vi "writeToXML.vi"(8 "error in (no error)":errorcluster, 10 "Class Label":string="WavefrontTargetPosition", 11 "WaveFrontTargetPosition in":refnum<class "WaveFrontTargetPosition.lvclass">) -> (0 "error out":errorcluster, 2 "XMLout":string, 3 "WaveFrontTargetPosition out":refnum<class "WaveFrontTargetPosition.lvclass">)   [LabVIEW 2022 SP3, in "TCSDataDefinitions.lvlib" / "TCSWFSStatus.lvlib" / "WaveFrontTargetPosition.lvclass"]
uses:
  WaveFrontTargetPosition.lvclass
  WaveFrontTargetPosition.lvclass/WaveFrontTargetPosition.ctl
  TCSWFSStatus/TCSWFSStatus.lvclass
  TCSGuiderStatus/GWTargetPositionParameters/GWTargetPositionParameters.lvclass
  <userlib>/Common/XML/XMLGenerator/XMLGenerator.lvclass
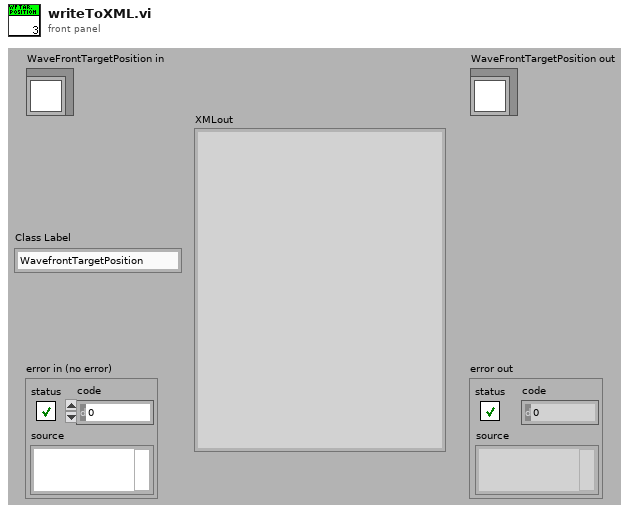
[diagram p1: front panel]
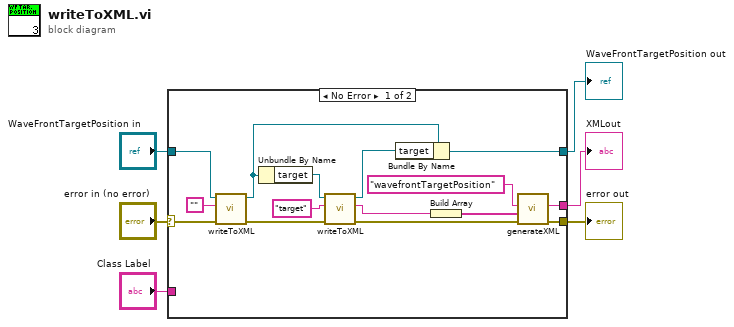
[diagram p0: block diagram]
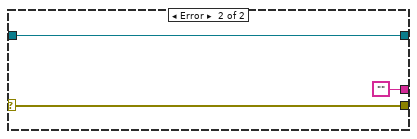
[diagram p2: hidden frame]
diagram:
  n1 = case shown="No Error" "error in (no error)" {
    selector: "error in (no error)" -> [w20 w24]
    tunnel: [w10 w24] -> w5
    tunnel: [w16 w23] -> w3
    tunnel: "WaveFrontTargetPosition in" -> [w21 w23]
    tunnel: [w9 ""] -> w2
    tunnel: "Class Label" -> [_ _]
    frame No Error {
      n2 = call-parent "writeToXML.vi"("error in (no error)"=w20, "ClassLabel"="", "TCSWFSStatus in"=w21) -> ("error out"=w15:errorcluster, "TCSWFSStatus out"=w18:refnum<class "WaveFrontTargetPosition.lvclass">)  [unwired: 6 in, 1 out]
      n3 = Unbundle By Name(w18) -> ("target"=w19:refnum<class "GWTargetPositionParameters.lvclass">)
      n4 = call-dynamic "writeToXML.vi"("error in (no error)"=w15, "Class Label"="target", "GWTargetPositionParameters in"=w19) -> ("error out"=w11:errorcluster, "outputXMLString"=w13:string, "GWTargetPositionParameters out"=w17:refnum<class "GWTargetPositionParameters.lvclass">)  [unwired: 6 in]
      n5 = Bundle By Name(cluster=w18, "target"=w17) -> (w16:refnum<class "WaveFrontTargetPosition.lvclass">)
      n6 = Build Array(w13) -> (w12:string[])
      n7 = call <userlib>:"generateXML.vi"("error in"=w11, "childrenXML"=w12, "elementName"="wavefrontTargetPosition" ("Class Label")) -> ("error out"=w10:errorcluster, "XML out"=w9:string)  [unwired: 6 in, 1 out]
    }
    frame Error {
    }
  }
  "error out" <- w5
  "WaveFrontTargetPosition out" <- w3
  "XMLout" <- w2
